vi "MM9.empty status string.vi"() -> (0 "String":string)   [LabVIEW 2014, in "MM9.lvlib"]
doc: "Just returns an empty string (of the right size) required for the \"Status\" service."
uses:
  MM9.lvlib
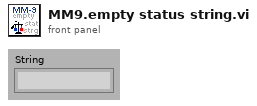
[diagram p1: front panel]
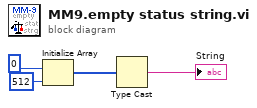
[diagram p0: block diagram]
diagram:
  n1 = Initialize Array(i8 0, 512 ("dimension size")) -> (w2:i8[])
  n2 = Type Cast(x=w2) -> (*(type *) &x=→"String":string)  [unwired: 1 in]
